vi "Get all info.vi"(8 "error in (no error)":errorcluster, 11 "VISA Refnum in":refnum<visa-resource-name>) -> (0 "error out":errorcluster, 2 "Recibo de Datos":string, 3 "VISA Refnum out":refnum<visa-resource-name>)   [LabVIEW 2020, in "Control de MaP.lvlib"]
uses:
  Control de MaP.lvlib
  Write--command.vi
  <vilib>/Instr/_visa.llb/VISA Flush IO Buffer Mask.ctl
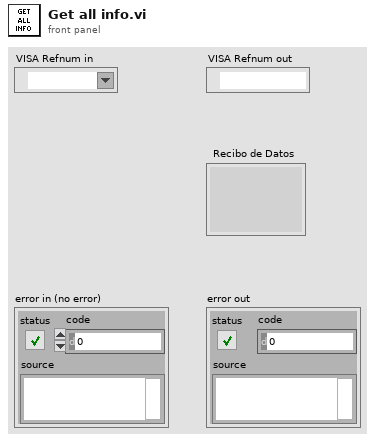
[diagram p1: front panel]
types:
  T1 = typedef "VISA Flush IO Buffer Mask.ctl" = u16
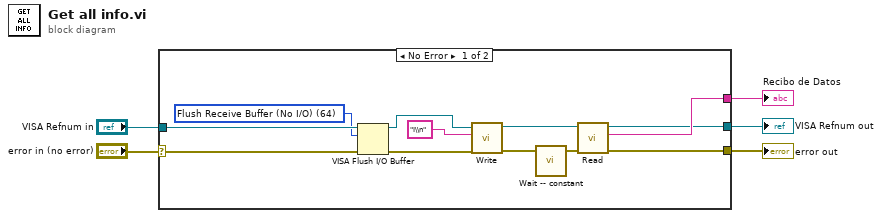
[diagram p0: block diagram]
diagram:
  n1 = case shown="No Error" "error in (no error)" {
    selector: "error in (no error)" -> [w13 w19]
    tunnel: [w17 _] -> w5
    tunnel: [w16 w18] -> w4
    tunnel: "VISA Refnum in" -> [w15 w18]
    tunnel: [w14 w19] -> w2
    frame No Error {
      w11 = T1 64 items=["Flush Receive Buffer"=16, "Write Transmit Buffer to Device"=32, "Flush Receive Buffer (No I/O)"=64, "Flush Transmit Buffer"=128] ("Mask")
      n2 = VISA Flush I/O Buffer(VISA resource name=w15, mask (16)=w11, error in (no error)=w13) -> (VISA resource name out=w9:refnum<visa-resource-name>, error out=w10:errorcluster)
      n3 = call-poly "Write.vi"("error in (no error)"=w10, "Command"="I\\n", "VISA resource name"=w9) -> ("error out"=w6:errorcluster, "VISA resource name out"=w8:refnum<visa-resource-name>)  [unwired: 6 in, 1 out]
      n4 = call "Wait -- constant.vi"("error in (no error)"=w6) -> ("error out"=w7:errorcluster)  [unwired: 4 in]
      n5 = call "Read.vi"("error in (no error)"=w7, "VISA resource name"=w8) -> ("error out"=w14:errorcluster, "Recibo de Datos"=w17:string, "VISA resource name out"=w16:refnum<visa-resource-name>)  [unwired: 6 in, 1 out]
    }
    frame Error {
    }
  }
  "Recibo de Datos" <- w5
  "VISA Refnum out" <- w4
  "error out" <- w2
